vi "RunReentrantViDynamically.vi"(8 "error in":errorcluster, 11 "ViRefIn":refnum<vi>) -> (0 "error out":errorcluster, 2 "VIName":string, 3 "ViRefNum":refnum<vi>)   [LabVIEW 2020]
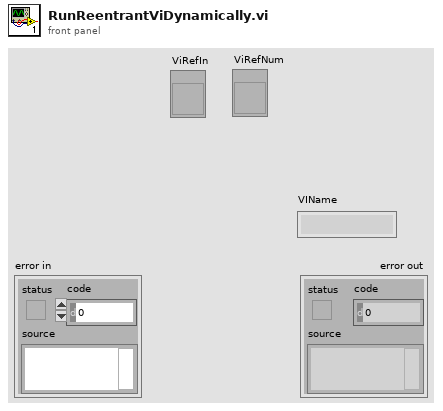
[diagram p1: front panel]
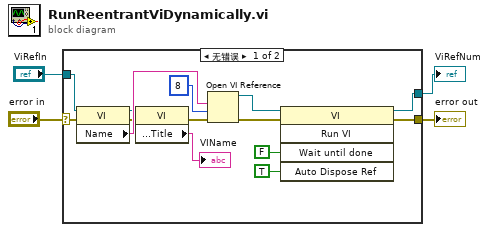
[diagram p0: block diagram]
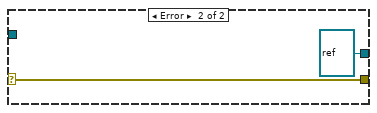
[diagram p2: hidden frame]
diagram:
  n1 = case shown="无错误" "error in" {
    selector: "error in" -> [w7 w20]
    tunnel: [w12 w20] -> w3
    tunnel: [w13 refnum<vi> refnum ("vi reference")] -> w2
    tunnel: "ViRefIn" -> [w10 _]
    frame No Error {
      n2 = property class="VI"(reference=w10, error in=w7) -> (reference out=w9:refnum<vi>, error out=w6:errorcluster, "Name"=w11:string)
      n3 = property class="VI"(reference=w9, error in=w6) -> (error out=w5:errorcluster, "Front Panel.Title"=→"VIName":string)  [unwired: 1 out]
      n4 = Open VI Reference(vi path=w11, options=8, error in (no error)=w5) -> (vi reference=w16:refnum<vi>, error out=w15:errorcluster)  [unwired: 3 out]
      n5 = invoke class="VI" method="Run VI"(reference=w16, error in=w15, "Wait until done"=FALSE ("Wait Until Done"), "Auto Dispose Ref"=TRUE ("Auto Dispose Reference")) -> (reference out=w13:refnum<vi>, error out=w12:errorcluster)  [unwired: 1 in, 3 out]
    }
    frame Error {
    }
  }
  "error out" <- w3
  "ViRefNum" <- w2
